vi "parse_laser_command.vi"(10 "Input String":string) -> (2 "Output String":string)   [LabVIEW 2023]
uses:
  Sirah_controls_2.6/LabVIEW/Laser/Laser Library LabVIEW 7.1/Laser Position Mode.ctl
  Sirah_controls_2.6/LabVIEW/Laser/Laser Library LabVIEW 7.1/Stage Reference.ctl
  <vilib>/regexp/Match Regular Expression.xnode
panel:
  out "error out":errorcluster
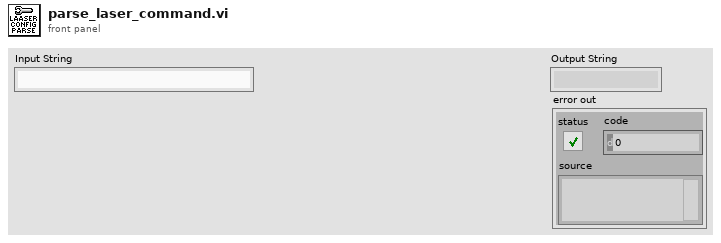
[diagram p1: front panel]
types:
  T1 = typedef "Laser Position Mode.ctl" = enum16{"fundamental, wavelength / nm", "fundamental, wavenumber / cm-1", "fundamental, frequency / GHz", "SHG, wavelength / nm", "SHG, wavenumber /  cm-1", "SHG, frequency / GHz", "DFM @ 1064 nm, wavelength / nm", "DFM @ 1064 nm, wavenumber / cm-1", "DFM @ 1064 nm, freuency / GHz", "OPA @ 1064 nm, wavelength / nm", "OPA @ 1064 nm, wavenumber / cm-1", "OPA @ 1064 nm, frequency / GHz", "THG, wavelength / nm", "THG, wavenumber / cm-1", "THG, frequency / GHz", "SFM @ 1064 nm, wavelength / nm", "SFM @ 1064 nm, wavenumber / cm-1", "SFM @ 1064 nm, frequency / GHz", "SFM @ 532 nm, wavelength / nm", "SFM @ 532 nm, wavenumber / cm-1", "SFM @ 532 nm, frequency / GHz", "SFM @ 355 nm, wavelength / nm", "SFM @ 355 nm, wavenumber / cm-1", "SFM @ 355 nm, frequency / GHz", "SFM @ 266 nm, wavelength / nm", "SFM @ 266 nm, wavenumber / cm-1", "SFM @ 266 nm, frequency / GHz", "NIR, wavelength / nm", "NIR, wavenumber / cm-1", "NIR, frequency / GHz", "DFM @ 355 nm, wavelength / nm", "DFM @ 355 nm, wavenumber / cm-1", "DFM @ 355 nm, frequency / GHz", "MAD @ 1064 nm, wavelength / nm", "MAD @ 1064 nm, wavenumber / cm-1", "MAD @ 1064 nm, frequency / GHz"}
  T2 = typedef "Stage Reference.ctl" = enum16{"Resonator", "Conversion(1)", "Conversion(2)", "Conversion(3)", "Conversion(4)", "Conversion(5)", "Conversion(6)", "Conversion(7)"}
  T3 = typedef "Laser Reference.ctl" = refnum<k4>
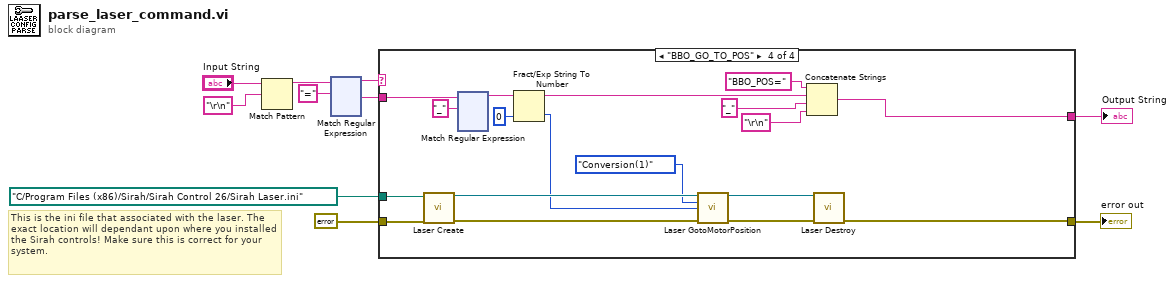
[diagram p0: block diagram]
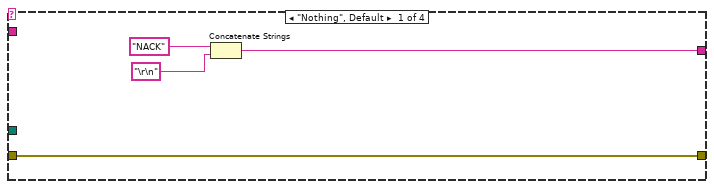
[diagram p2: hidden frame]
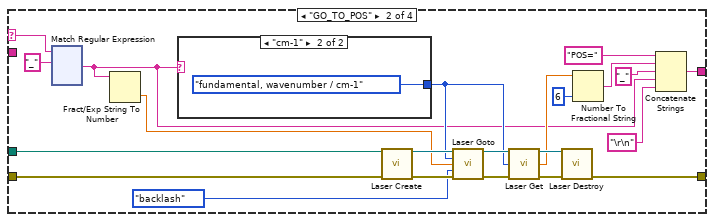
[diagram p3: hidden frame]
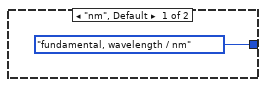
[diagram p4: hidden frame]
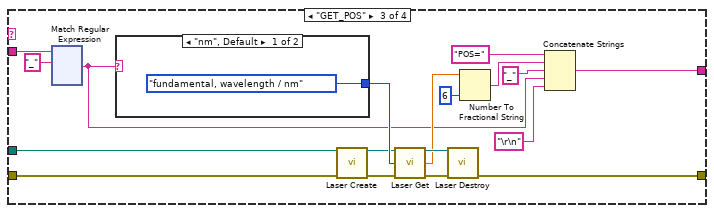
[diagram p5: hidden frame]
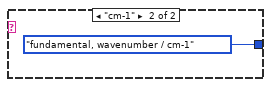
[diagram p6: hidden frame]
diagram:
  # "This is the ini file that associated with the laser. The exact location will dependant upon where you installed the Sirah controls! Make sure this is correct for your system."
  n1 = Match Pattern(string="Input String", regular expression="\r\n") -> (before substring=w2:string)  [unwired: 1 in, 3 out]
  n2 = xnode "Match Regular Expression"("input string"=w2, "regular expression"="=") -> ("before match"=w7:string, "after match"=w1:string)  [unwired: 4 in, 3 out]
  n3 = case shown="\"BBO_GO_TO_POS\"" w7 {
    selector: w7 -> [_ w15 _ _]
    tunnel: [w14 w29 w171 w307] -> w4
    tunnel: errorcluster {"status"=FALSE, "code"=0, "source"=""} ("error in (no error)") -> [w14 w28 w170 w308]
    tunnel: path "C:/Program Files (x86)/Sirah/Sirah Control 26/Sirah Laser.ini" ("configuration filename") -> [_ w26 w168 w309]
    tunnel: [w13 w19 w161 w296] -> w3
    tunnel: w1 -> [_ _ w156 w301]
    frame "Nothing", Default {
      n4 = Concatenate Strings("NACK", "\r\n" ("regular expression")) -> (w13:string)
    }
    frame "GO_TO_POS" {
      n5 = xnode "Match Regular Expression"("input string"=w15, "regular expression"="_") -> ("after match"=w18:string)  [unwired: 4 in, 4 out]
      n6 = Fract/Exp String To Number(string=w18) -> (number=w17:dbl)  [unwired: 3 in, 1 out]
      n7 = case shown="\"cm-1\"" w18 {
        tunnel: [Laser_Position_Mode."fundamental, wavelength / nm" ("laser position mode (fundamental wavelength)") Laser_Position_Mode."fundamental, wavenumber / cm-1" ("laser position mode (fundamental wavelength)")] -> w27
        frame "nm", Default {
        }
        frame "cm-1" {
        }
      }
      n8 = call "Laser Create.vi"("configuration filename"=w26, "error in (no error)"=w28) -> ("laser out"=w36:T3, "error out"=w35:errorcluster)  [unwired: 12 in]
      n9 = call "Laser Goto.vi"("laser"=w36, "laser position mode (fundamental wavelength)"=w27, "position"=w17, "mode (backlash)"=enum16{"backlash", "no backlash"}."backlash", "error in (no error)"=w35) -> ("laser out"=w33:T3, "error out"=w32:errorcluster)  [unwired: 9 in]
      n10 = call "Laser Get.vi"("laser"=w33, "laser position mode (fundamental wavelength)"=w27, "error in (no error)"=w32) -> ("laser out"=w31:T3, "position"=w25:dbl, "error out"=w30:errorcluster)  [unwired: 10 in]
      n11 = call "Laser Destroy.vi"("laser"=w31, "error in (no error)"=w30) -> ("error out"=w29:errorcluster)  [unwired: 13 in]
      n12 = Number To Fractional String(number=w25, precision (6)=i16 6) -> (F-format string=w24:string)  [unwired: 2 in]
      n13 = Concatenate Strings("POS=", w24, "_" ("string"), w18, "\r\n" ("regular expression")) -> (w19:string)
    }
    frame "GET_POS" {
      n14 = xnode "Match Regular Expression"("input string"=w156, "regular expression"="_") -> ("after match"=w160:string)  [unwired: 4 in, 4 out]
      n15 = case shown="\"nm\", Default" w160 {
        tunnel: [Laser_Position_Mode."fundamental, wavelength / nm" ("laser position mode (fundamental wavelength)") Laser_Position_Mode."fundamental, wavenumber / cm-1" ("laser position mode (fundamental wavelength)")] -> w169
        frame "nm", Default {
        }
        frame "cm-1" {
        }
      }
      n16 = call "Laser Create.vi"("configuration filename"=w168, "error in (no error)"=w170) -> ("laser out"=w158:T3, "error out"=w157:errorcluster)  [unwired: 12 in]
      n17 = call "Laser Get.vi"("laser"=w158, "laser position mode (fundamental wavelength)"=w169, "error in (no error)"=w157) -> ("laser out"=w173:T3, "position"=w167:dbl, "error out"=w172:errorcluster)  [unwired: 10 in]
      n18 = call "Laser Destroy.vi"("laser"=w173, "error in (no error)"=w172) -> ("error out"=w171:errorcluster)  [unwired: 13 in]
      n19 = Number To Fractional String(number=w167, precision (6)=i16 6) -> (F-format string=w166:string)  [unwired: 2 in]
      n20 = Concatenate Strings("POS=", w166, "_" ("string"), w160, "\r\n" ("regular expression")) -> (w161:string)
    }
    frame "BBO_GO_TO_POS" {
      n21 = call "Laser Create.vi"("configuration filename"=w309, "error in (no error)"=w308) -> ("laser out"=w304:T3, "error out"=w303:errorcluster)  [unwired: 12 in]
      n22 = xnode "Match Regular Expression"("input string"=w301, "regular expression"="_") -> ("before match"=w294:string)  [unwired: 4 in, 4 out]
      n23 = Fract/Exp String To Number(string=w294, default (0 dbl)=0) -> (number=w298:i32)  [unwired: 2 in, 1 out]
      n24 = call "Laser GotoMotorPosition.vi"("laser"=w304, "stage ID"=Stage_Reference."Conversion(1)", "position"=w298, "error in (no error)"=w303) -> ("laser out"=w306:T3, "error out"=w305:errorcluster)  [unwired: 10 in]
      n25 = Concatenate Strings("BBO_POS=", w294, "_" ("string"), "\r\n" ("regular expression")) -> (w296:string)
      n26 = call "Laser Destroy.vi"("laser"=w306, "error in (no error)"=w305) -> ("error out"=w307:errorcluster)  [unwired: 13 in]
    }
  }
  "error out" <- w4
  "Output String" <- w3
